vi "Calculate Board Duration.vi"(10 "Board":i32[][](array[numeric]), 11 "Draw":i32[](array[numeric])) -> (0 "Marked":bool[][](array[boolean]), 1 "Index":i32, 2 "Row?":bool, 3 "Duration":i32)   [LabVIEW 2021]
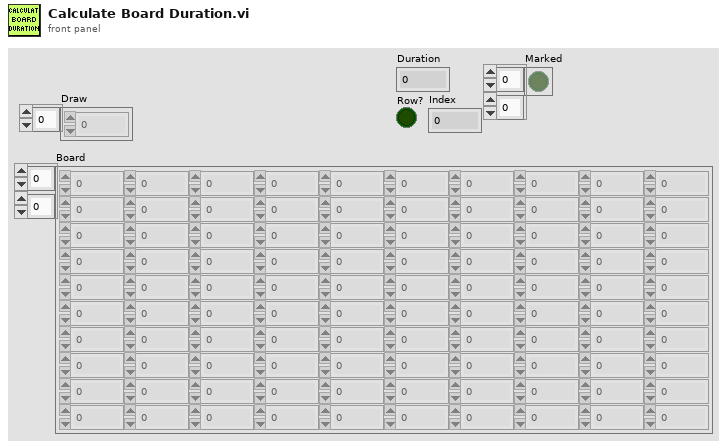
[diagram p1: front panel]
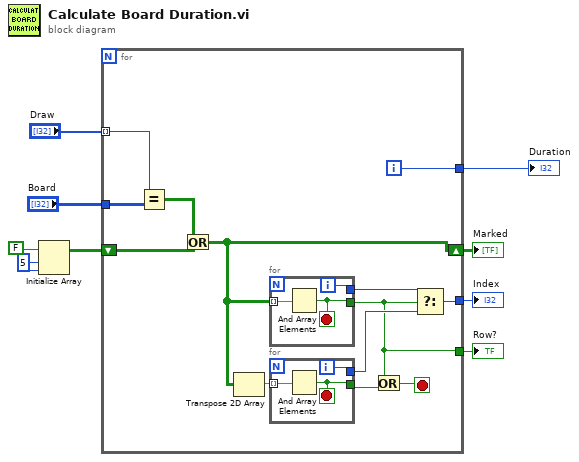
[diagram p0: block diagram]
diagram:
  w6 = 5 ("dimension size")
  n1 = Initialize Array(FALSE, w6, w6) -> (w5:bool[][])
  n2 = for {
    tunnel: "Board" -> [w22]
    tunnel: "Draw" -> [w21] mode=indexing
    shift-right: [w17] -> w1
    shift-left: w5 -> [w20]
    tunnel: [w14] -> w4
    tunnel: [w11] -> w2
    tunnel: [w10] -> w3
    i -> [w14]
    stop <- w15 stop-if-true
    n3 = Equal?(x=w21, y=w22) -> (x = y?=w19:bool[][])
    n4 = Or(x=w19, y=w20) -> (x .or. y?=w17:bool[][])
    n5 = Transpose 2D Array(2D array=w17) -> (transposed array=w18:bool[][])
    n6 = for {
      tunnel: w17 -> [w28] mode=indexing
      tunnel: [w27] -> w10
      tunnel: [w26] -> w13
      i -> [w26]
      stop <- w27 stop-if-true
      n7 = And Array Elements(Boolean array=w28) -> (logical AND=w27:bool)
    }
    n8 = for {
      tunnel: w18 -> [w25] mode=indexing
      tunnel: [w24] -> w16
      tunnel: [w23] -> w12
      i -> [w23]
      stop <- w24 stop-if-true
      n9 = And Array Elements(Boolean array=w25) -> (logical AND=w24:bool)
    }
    n10 = Or(x=w10, y=w16) -> (x .or. y?=w15:bool)
    n11 = Select(t=w13, s=w10, f=w12) -> (s? t:f=w11:i32)
  }
  "Duration" <- w4
  "Row?" <- w3
  "Index" <- w2
  "Marked" <- w1
